vi "FGV SPAN Stufentabellen.vi"(5 "Aktion":T3, 7 "error in (no error)":errorcluster caption="Fehler (Eingang, kein Fehler)", 10 "In Cluster":T2) -> (0 "error out":errorcluster caption="Fehler (Ausgang)", 1 "EGAK Arrays":string[][](array[string]), 2 "SPAN Stufentabellen":string[][][][](array[string]), 3 "Out Cluster":T2)   [LabVIEW 2020, in "Linearisierung v2.lvlib" / "SpanEinstellungen.lvlib"]
uses:
  SpanEinstellungen.lvlib
  Aktion FGV SPAN Stufentabellen.ctl
  Gasteiler/Stufen Tabelle.ctl
  Linearisierung v2.lvlib
  Gasteiler/Gasteiler.lvlib
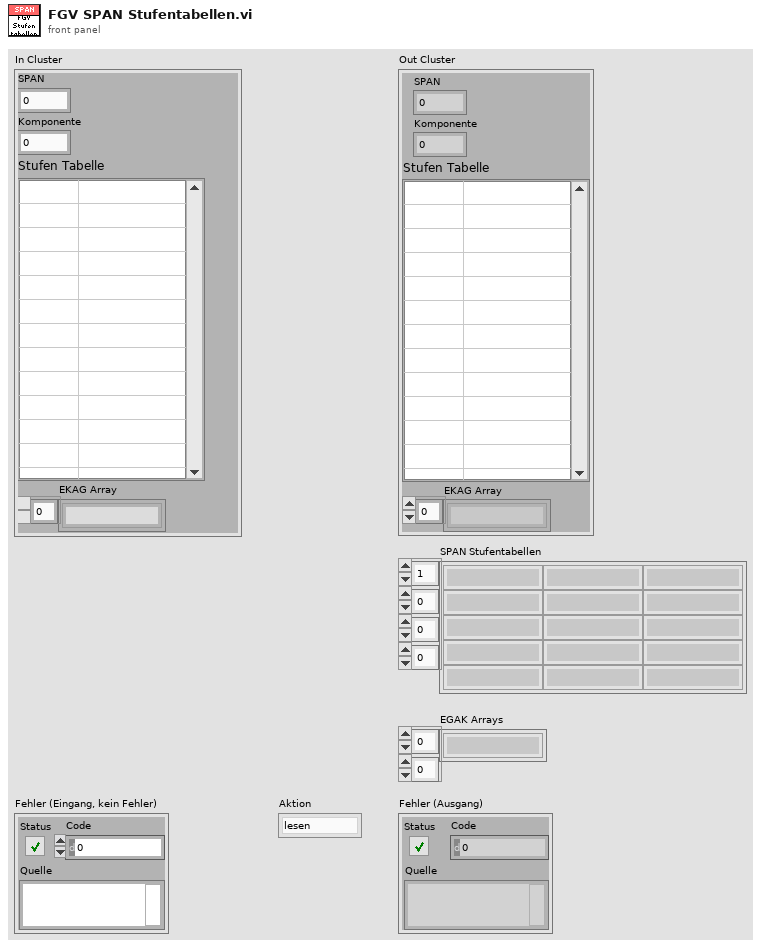
[diagram p1: front panel]
types:
  T1 = typedef "Linearisierung v2.lvlib/Gasteiler.lvlib/Stufen Tabelle.ctl" = string[][]
  T2 = cluster{"SPAN":i32, "Komponente":i32, "Stufen Tabelle":T1, "EKAG Array":string[]}
  T3 = typedef "Linearisierung v2.lvlib/SpanEinstellungen.lvlib/Aktion FGV SPAN Stufentabellen.ctl" = enum16{"lesen", "schreiben", "init"}
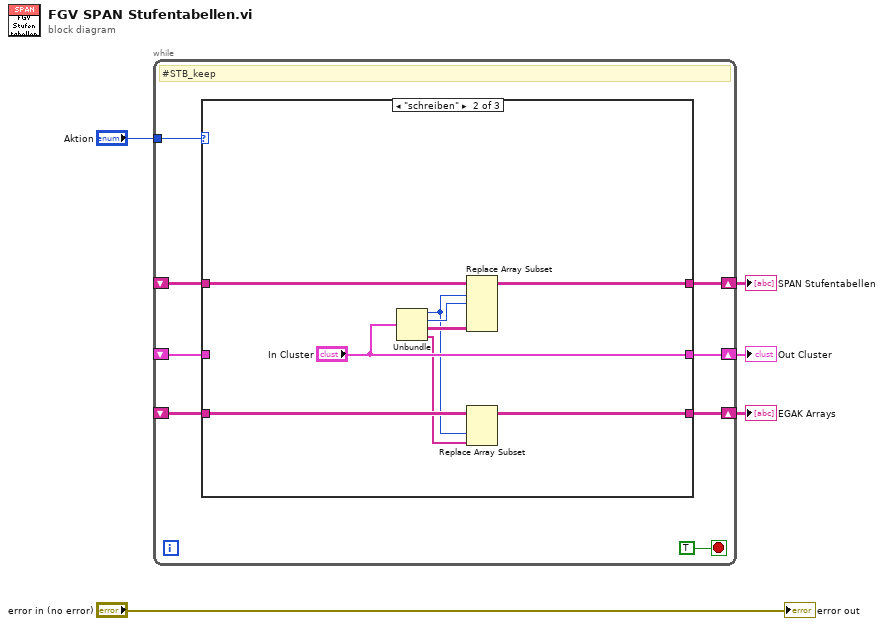
[diagram p0: block diagram]
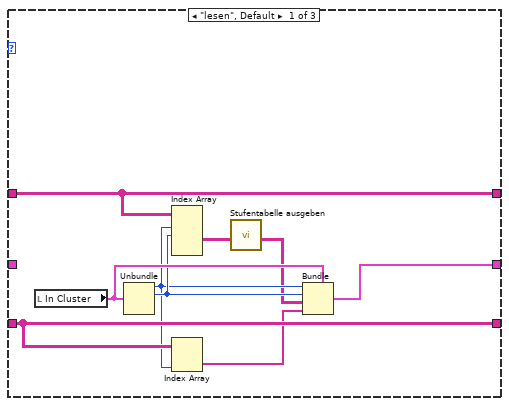
[diagram p2: hidden frame]
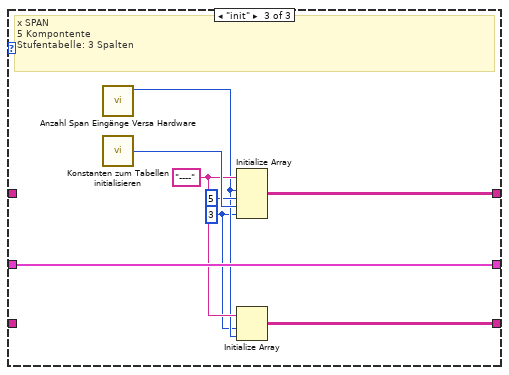
[diagram p3: hidden frame]
diagram:
  n1 = while {
    tunnel: "Aktion" -> [w13]
    shift-right: [w11] -> w3
    shift-left: _ -> [w10]
    shift-right: [w9] -> w2
    shift-left: _ -> [w8]
    shift-right: [w7] -> w1
    shift-left: _ -> [w6]
    stop <- TRUE stop-if-true
    # "#STB_keep"
    n2 = case shown="\"schreiben\"" w13 {
      tunnel: [w22 w30 w39] -> w11
      tunnel: w10 -> [w22 w31 _]
      tunnel: [w20 "In Cluster" w36] -> w9
      tunnel: w8 -> [_ _ w36]
      tunnel: [w18 w25 w35] -> w7
      tunnel: w6 -> [w18 w26 _]
      frame "lesen", Default {
        n3 = local read "In Cluster"() -> (w21:T2)
        n4 = Unbundle(w21) -> ("SPAN"=w16:i32, "Komponente"=w19:i32)  [unwired: 2 out]
        n5 = Index Array(array=w22, index (dim 0)=w16, index (dim 1)=w19) -> (element=w15:string[][])  [unwired: 2 in]
        n6 = Index Array(array=w18, index (col)=w16) -> (element=w17:string[])  [unwired: 1 in]
        n7 = call "Stufentabelle ausgeben.vi"("Neue Tabelle"=w15) -> ("Tabelle"=w14:string[][])  [unwired: 10 in]
        n8 = Bundle(cluster=w21, "SPAN"=w16, "Komponente"=w19, "Stufen Tabelle"=w14, "EKAG Array"=w17) -> (w20:T2)
      }
      frame "schreiben" {
        n9 = Unbundle("In Cluster") -> ("SPAN"=w24:i32, "Komponente"=w28:i32, "Stufen Tabelle"=w27:T1, "EKAG Array"=w23:string[])
        n10 = Replace Array Subset(array=w31, new element=w27, index (dim 0)=w24, index (dim 1)=w28) -> (w30:string[][][][])  [unwired: 2 in]
        n11 = Replace Array Subset(array=w26, new element=w23, index (col)=w24) -> (w25:string[][])  [unwired: 1 in]
      }
      frame "init" {
        w32 = 3 ("Dimension")
        w34 = "----"
        # "x SPAN\n5 Kompontente\nStufentabelle: 3 Spalten"
        n12 = call "Anzahl Span Eingänge Versa Hardware.vi"() -> ("Anzahl Span"=w33:i32)  [unwired: 11 in]
        n13 = call "Konstanten zum Tabellen initialisieren.vi"() -> ("Anzahl Tabellenzeilen"=w38:i32)  [unwired: 13 in, 2 out]
        n14 = Initialize Array(w34, w33, 5 ("Dimensionsgröße"), w38, w32) -> (w39:string[][][][])
        n15 = Initialize Array(w34, w32, w33) -> (w35:string[][])
      }
    }
  }
  "SPAN Stufentabellen" <- w3
  "Out Cluster" <- w2
  "EGAK Arrays" <- w1
  "error out" <- "error in (no error)"
